vi "Sample - Job Record (SubVI).vi"(8 "error in":errorcluster) -> (0 "error out":errorcluster)   [LabVIEW 2019]
uses:
  Controls/Job record-state.ctl
  Controls/JSON - Job.ctl
  <vilib>/httpClient/POSTBuffer.vi
  <vilib>/httpClient/LabVIEWHTTPClient.lvlib
panel:
  in  "Please select Job No to delete":u16(ring) items=["GS1", "GS2"]
  in  "Ok":bool
  in  "Delete":bool
  out "TABLE":string[][](table)
  in  "Add":bool
  in  "Job Description":string
  in  "Job No":string
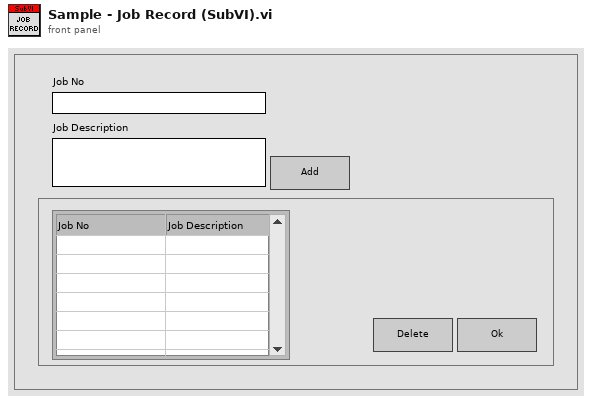
[diagram p1: front panel]
types:
  T1 = typedef "Job record-state.ctl" = enum16{"Init", "Read DB", "Idle", "update", "delete", "close"}
  T2 = typedef "JSON - Job.ctl" = cluster{"status":string, "data":cluster{"id":string, "jobno":string, "jobdesc":string, "delete":string, "created_date":string}[]}
  T3 = cluster{"action":string, "jobno":string, "jobdesc":string}
  T4 = cluster{"Jobs No":string, "Key Value":string[]}[]
  T5 = typedef "LabVIEWHTTPClient.lvlib/ClientHandle.ctl" = refnum<k1>
  T6 = cluster{"id":string, "jobno":string, "jobdesc":string, "delete":string, "created_date":string}[]
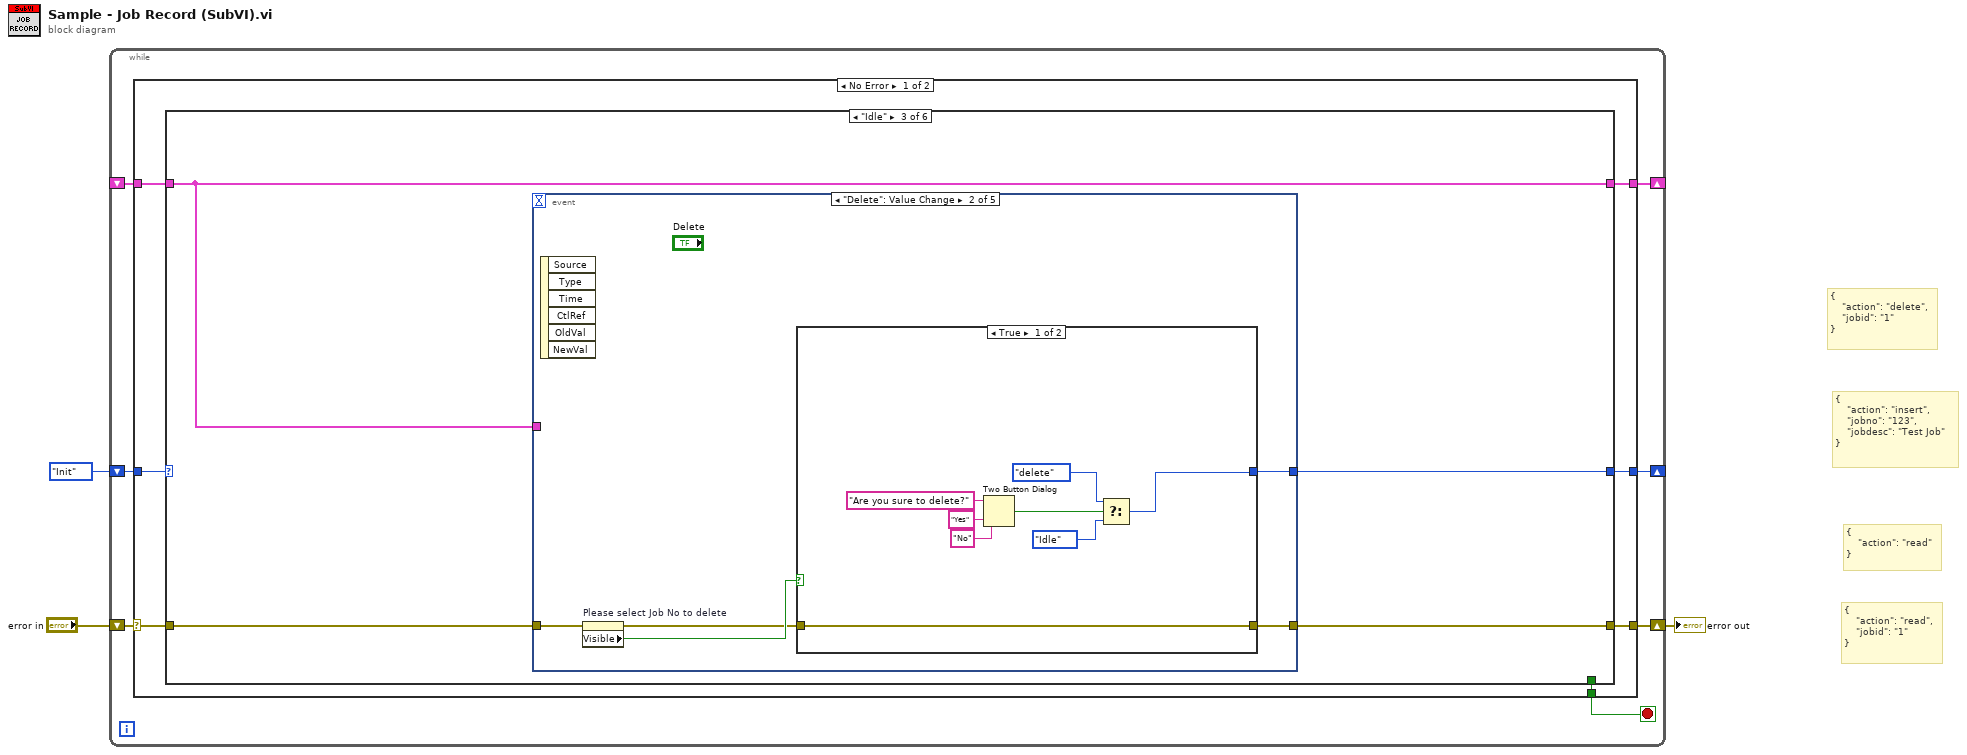
[diagram p0: block diagram]
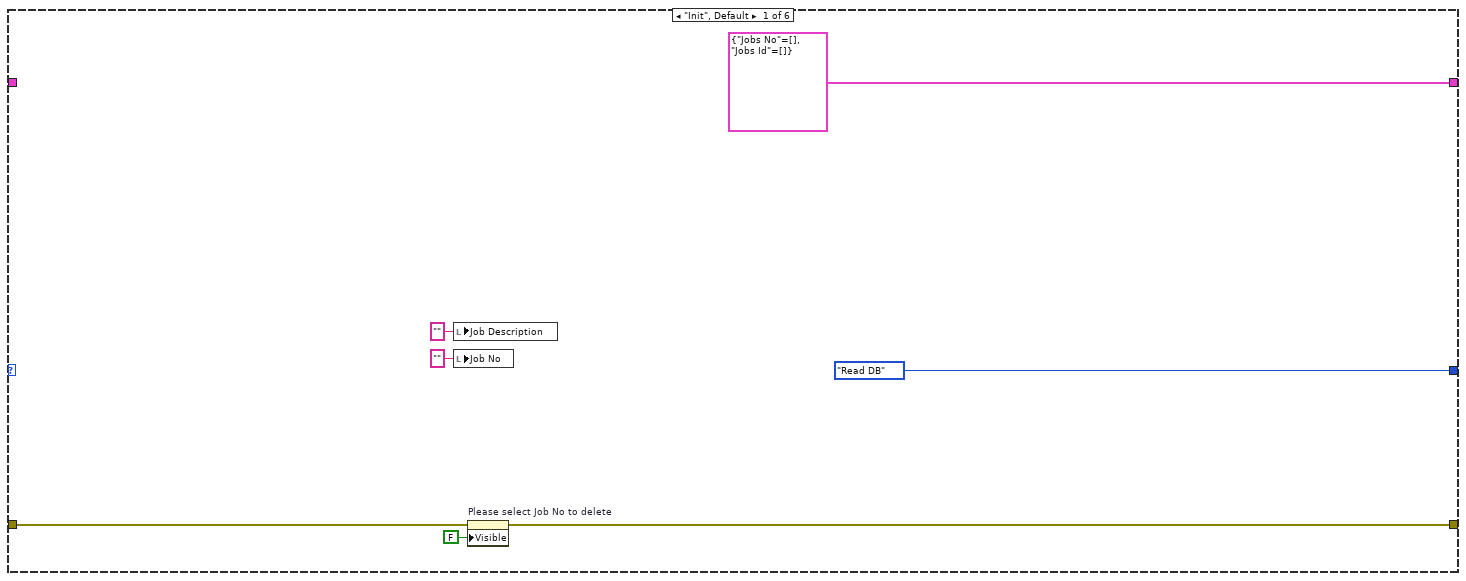
[diagram p2: hidden frame]
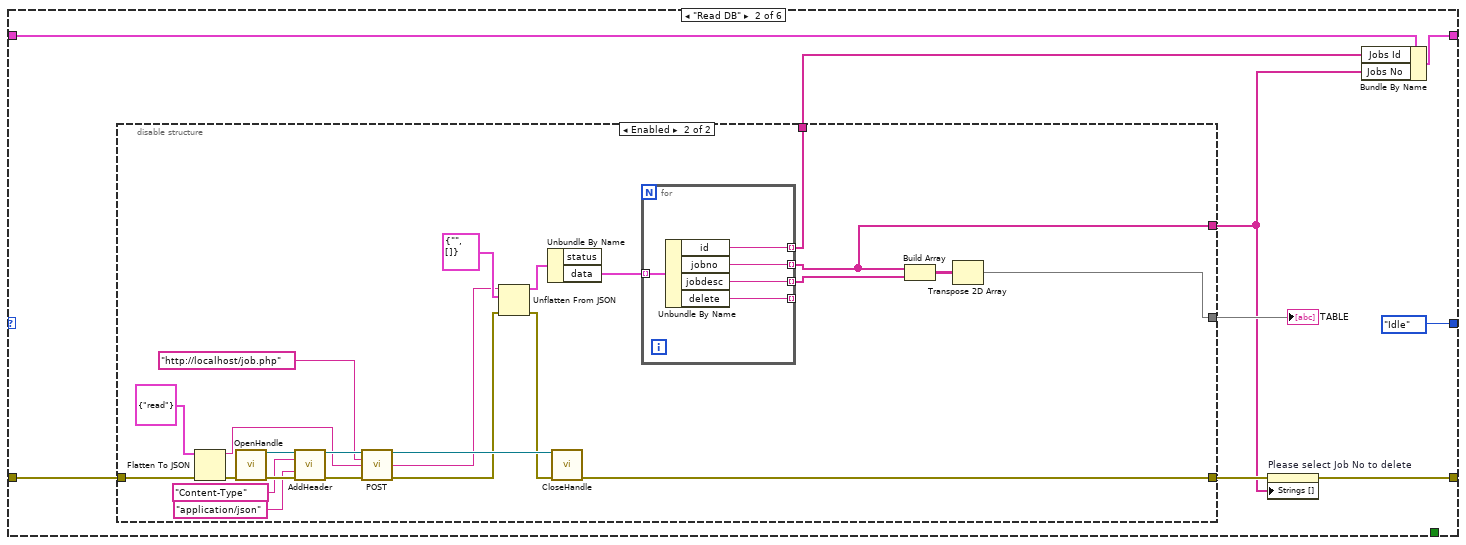
[diagram p3: hidden frame]
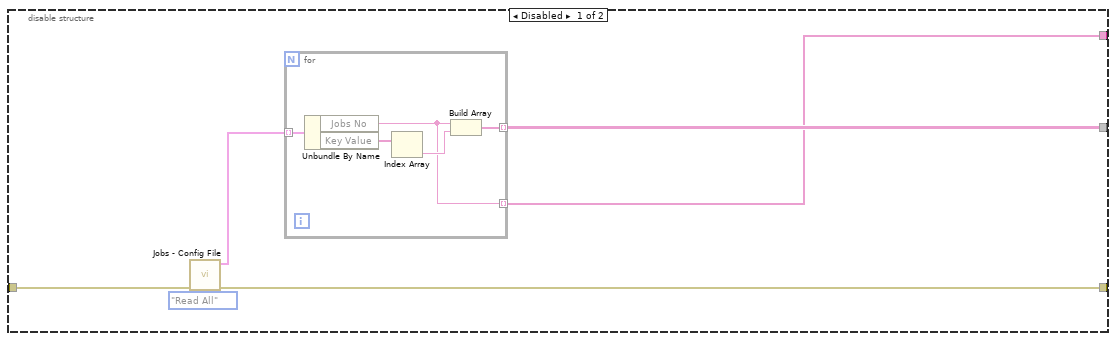
[diagram p4: hidden frame]
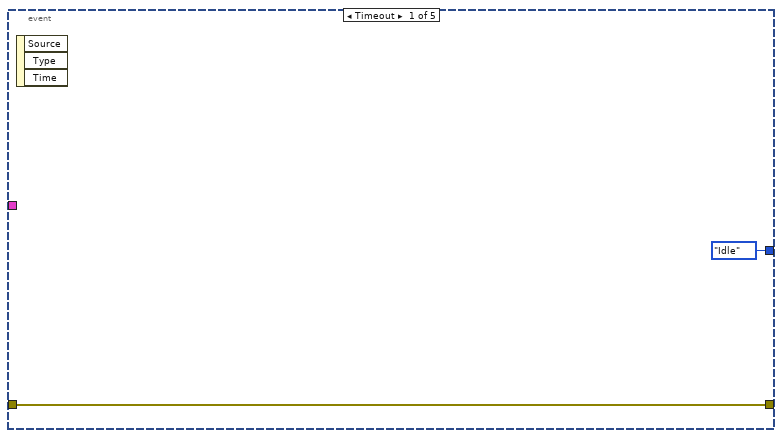
[diagram p5: hidden frame]
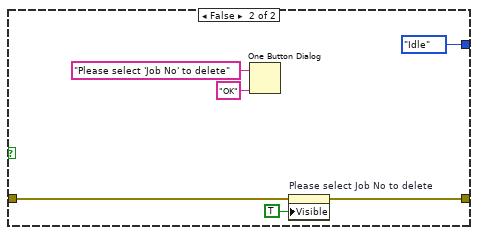
[diagram p6: hidden frame]
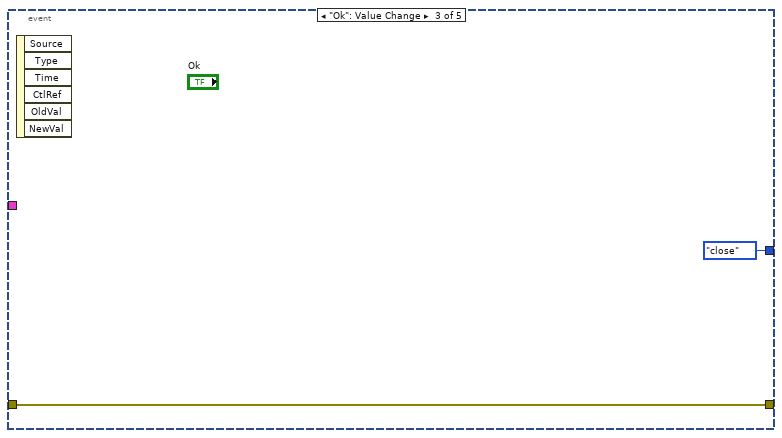
[diagram p7: hidden frame]
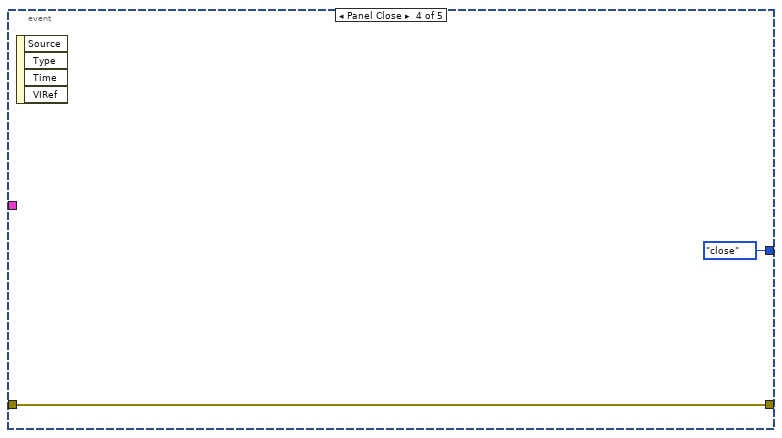
[diagram p8: hidden frame]
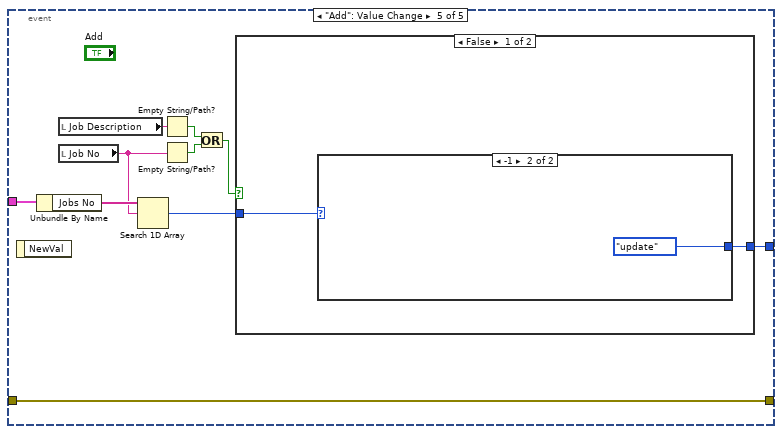
[diagram p9: hidden frame]
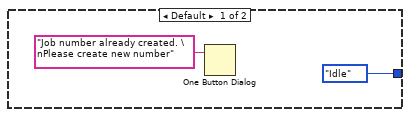
[diagram p10: hidden frame]
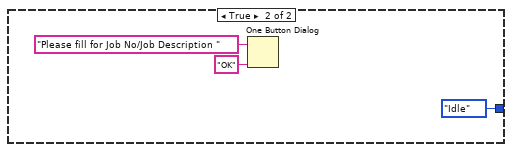
[diagram p11: hidden frame]
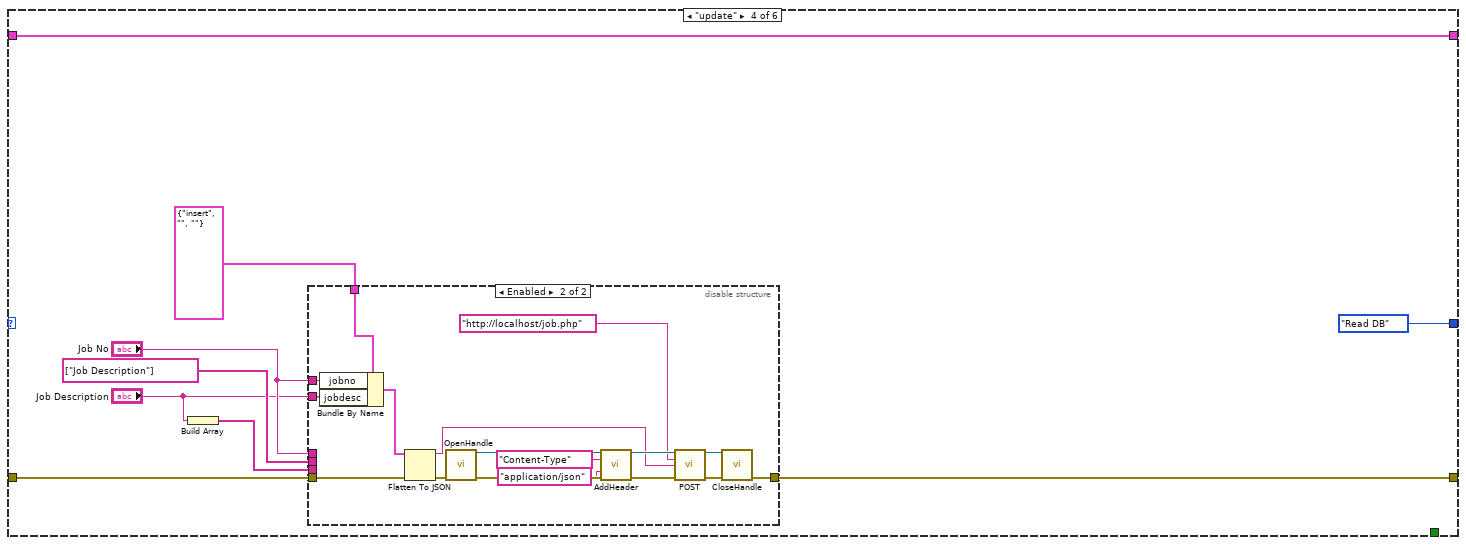
[diagram p12: hidden frame]
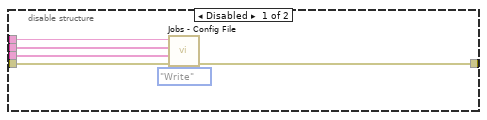
[diagram p13: hidden frame]
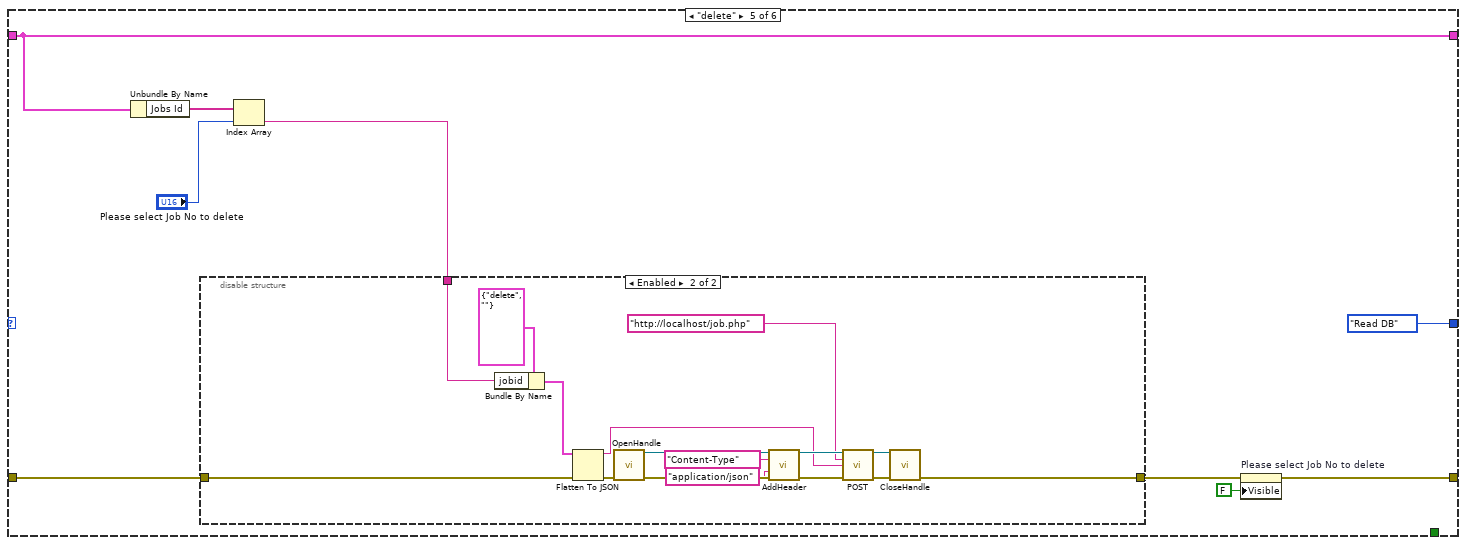
[diagram p14: hidden frame]
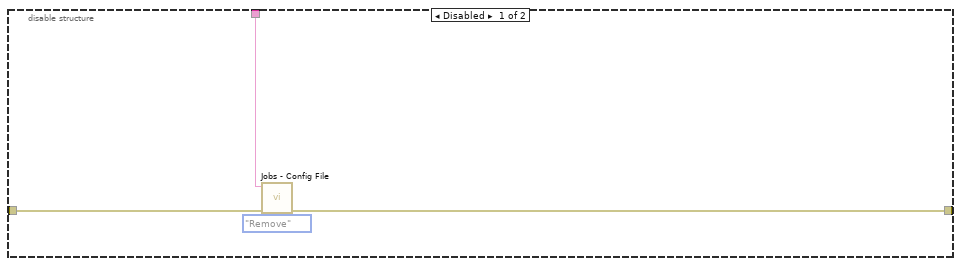
[diagram p15: hidden frame]
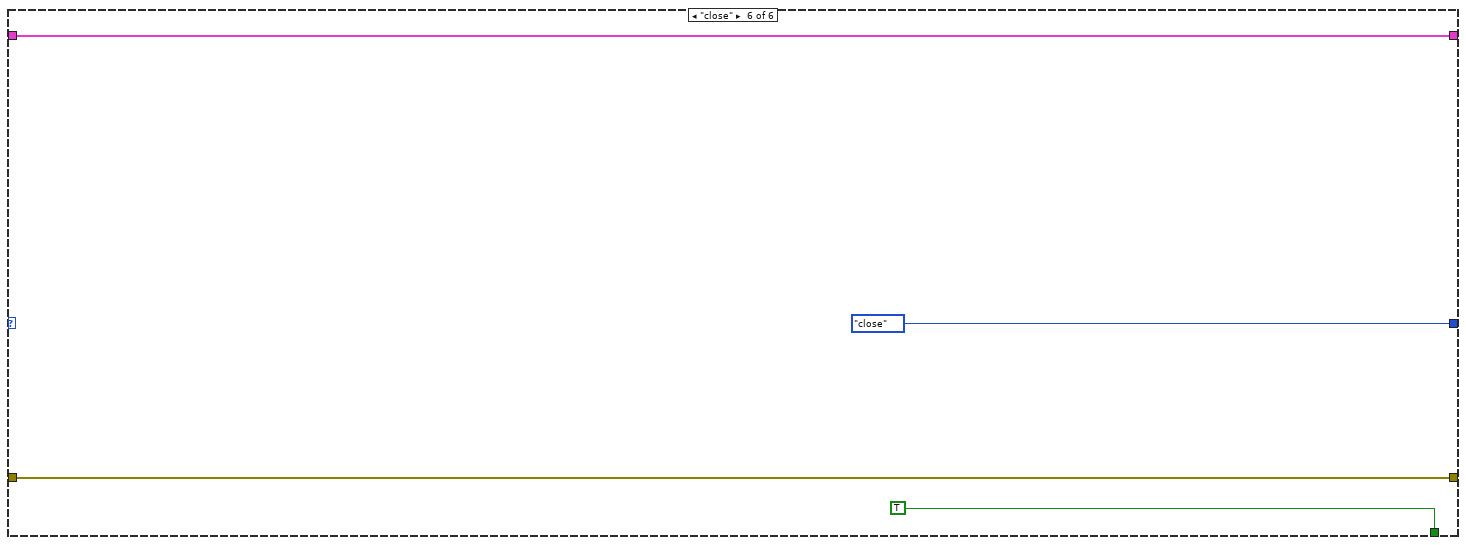
[diagram p16: hidden frame]
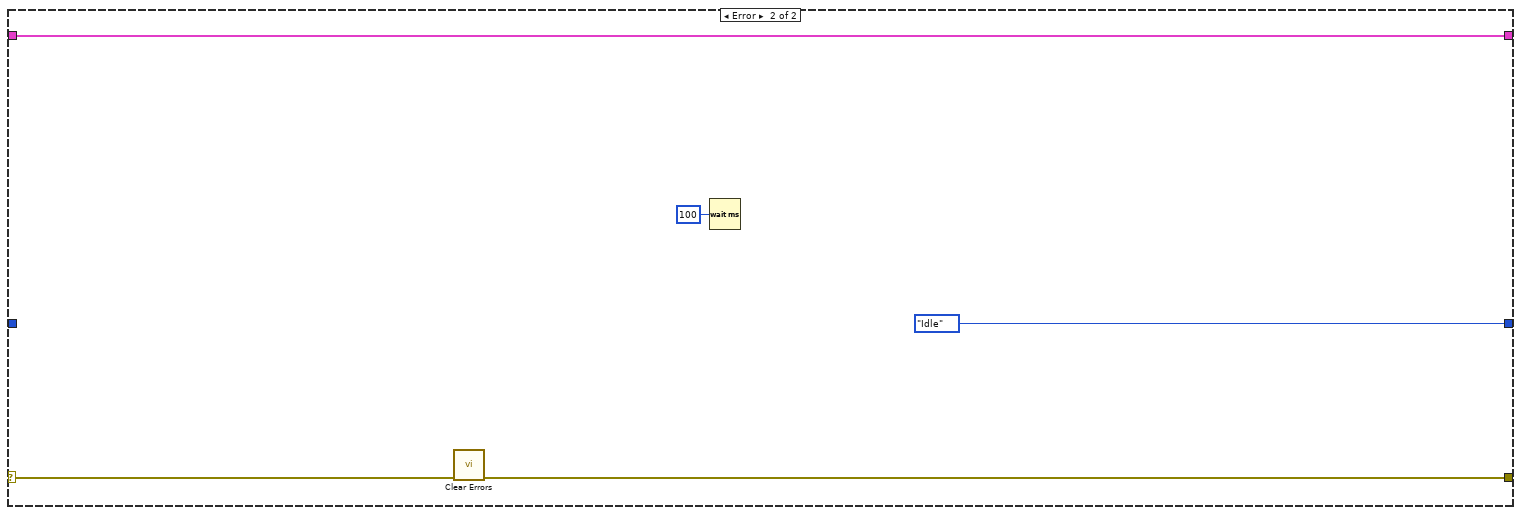
[diagram p17: hidden frame]
diagram:
  # "{\n    \"action\": \"read\",\n    \"jobid\": \"1\"\n}"
  # "{\n    \"action\": \"read\"\n}"
  # "{\n    \"action\": \"delete\",\n    \"jobid\": \"1\"\n}"
  # "{\n    \"action\": \"insert\",\n    \"jobno\": \"123\",\n    \"jobdesc\": \"Test Job\"\n}"
  n1 = while {
    shift-right: [w8] -> w1
    shift-left: "error in" -> [w10]
    shift-right: [w7] -> _
    shift-left: Job_record-state."Init" -> [w9]
    shift-right: [w6] -> _
    shift-left: _ -> [w5]
    stop <- w4 stop-if-true
    n2 = case shown="No Error" w10 {
      selector: w10 -> [w17 w190]
      tunnel: w9 -> [w16 _]
      tunnel: [w15 w189] -> w8
      tunnel: [w14 Job_record-state."Idle"] -> w7
      tunnel: [w13 w186] -> w6
      tunnel: w5 -> [w12 w186]
      tunnel: [w11 _] -> w4
      frame No Error {
        n3 = case shown="\"Idle\"" w16 {
          tunnel: w17 -> [w18 w30 w77 w127 w155 w185]
          tunnel: [w19 w28 w76 w126 w157 w185] -> w15
          tunnel: [Job_record-state."Read DB" Job_record-state."Idle" w75 Job_record-state."Read DB" Job_record-state."Read DB" Job_record-state."close"] -> w14
          tunnel: [cluster{"Jobs No":string[], "Jobs Id":string[]} {"Jobs No"=[], "Jobs Id"=[]} w32 w74 w128 w161 w182] -> w13
          tunnel: w12 -> [_ w31 w74 w128 w161 w182]
          tunnel: [_ _ _ _ _ TRUE] -> w11
          frame "Init", Default {
            n4 = local write "Job Description"("" ("Job Description")) -> ()
            n5 = local write "Job No"("" ("Job No")) -> ()
            n6 = property on="Please select Job No to delete" class="Ring (strict)"(error in=w18, "Visible"=FALSE) -> (error out=w19:errorcluster)  [unwired: 1 in, 1 out]
          }
          frame "Read DB" {
            n7 = disable-structure shown="Enabled" {
              disable-tunnel: w30 -> [w38 w58]
              disable-tunnel: [w36 w57] -> w29
              disable-tunnel: [w35 w47] -> w27
              disable-tunnel: [w34 w45] -> w26
              disable-tunnel: [_ w46] -> w25
              frame Disabled {
                n8 = call "Jobs - Config File.vi"("Action"=enum16{"Write", "Read", "Read All", "Remove"}."Read All", "error in (no error)"=w38) -> ("error out"=w36:errorcluster, "Value Out"=w37:T4)  [unwired: 7 in, 1 out]
                n9 = for {
                  tunnel: w37 -> [w44] mode=indexing
                  tunnel: [w41] -> w35 mode=indexing
                  tunnel: [w40] -> w34 mode=indexing
                  n10 = Unbundle By Name(w44) -> ("Jobs No"=w40:string, "Key Value"=w43:string[])
                  n11 = Index Array(array=w43) -> (element=w42:string)  [unwired: 1 in]
                  n12 = Build Array(w40, w42) -> (w41:string[])
                }
              }
              frame Enabled {
                n13 = Flatten To JSON(anything=cluster{"action":string} {"action"="read"}, error in (no error)=w58) -> (JSON string=w62:string, 11:w63:errorcluster)  [unwired: 1 in]
                n14 = call <vilib>:"OpenHandle.vi"("error in (no error)"=w63) -> ("client handle out"=w66:T5, "error out"=w68:errorcluster)  [unwired: 13 in]
                n15 = call <vilib>:"AddHeader.vi"("client handle"=w66, "header"="Content-Type", "value"="application/json", "error in (no error)"=w68) -> ("client handle out"=w65:T5, "error out"=w67:errorcluster)  [unwired: 10 in]
                n16 = call-poly <vilib>:"POST.vi"("client handle"=w65, "url"="http://localhost/job.php", "buffer"=w62, "error in (no error)"=w67) -> ("client handle out"=w64:T5, "body"=w52:string, "error out"=w51:errorcluster)  [unwired: 8 in, 1 out]
                n17 = Unflatten From JSON(JSON string=w52, type and defaults=T2 {"status"="", "data"=[]}, error in (no error)=w51) -> (value=w54:T2, error out=w50:errorcluster)  [unwired: 4 in]
                n18 = Unbundle By Name(w54) -> ("data"=w53:T6)  [unwired: 1 out]
                n19 = call <vilib>:"CloseHandle.vi"("client handle"=w64, "error in (no error)"=w50) -> ("error out"=w57:errorcluster)  [unwired: 13 in]
                n20 = for {
                  tunnel: w53 -> [w73] mode=indexing
                  tunnel: [w72] -> w46 mode=indexing
                  tunnel: [w71] -> w45 mode=indexing
                  tunnel: [w70] -> w49 mode=indexing
                  tunnel: [w69] -> _ mode=indexing
                  n21 = Unbundle By Name(w73) -> ("id"=w72:string, "jobno"=w71:string, "jobdesc"=w70:string, "delete"=w69:string)
                }
                n22 = Build Array(w45, w49) -> (w48:string[][])
                n23 = Transpose 2D Array(2D array=w48) -> (transposed array=w47:string[][])
              }
            }
            "TABLE" <- w27
            n24 = property on="Please select Job No to delete" class="Ring (strict)"(error in=w29, "Strings []"=w26) -> (error out=w28:errorcluster)  [unwired: 1 in, 1 out]
            n25 = Bundle By Name(cluster=w31, "Jobs Id"=w25, "Jobs No"=w26) -> (w32:cluster{"Jobs No":string[], "Jobs Id":string[]})
          }
          frame "Idle" {
            n26 = event shown="[1] \"Delete\": Value Change" {
              selector: _ -> [_ _ _ _ _]
              dyn-events: _ -> [_ _ _ _ _]
              timeout: _ -> [_ _ _ _ _]
              tunnel: [w79 w82 w99 w101 w112] -> w76
              tunnel: w77 -> [w79 w80 w99 w101 w112]
              tunnel: [Job_record-state."Idle" w84 Job_record-state."close" Job_record-state."close" w111] -> w75
              tunnel: w74 -> [_ _ _ _ w106]
              event Timeout {
                n27 = event-data() -> ()  [unwired: 1 in, 3 out]
              }
              event "Delete": Value Change {
                n28 = event-data() -> ()  [unwired: 1 in, 6 out]
                n29 = property on="Please select Job No to delete" class="Ring (strict)"(error in=w80) -> (error out=w81:errorcluster, "Visible"=w83:bool)  [unwired: 1 in, 1 out]
                n30 = case shown="True" w83 {
                  tunnel: [w87 Job_record-state."Idle"] -> w84
                  tunnel: w81 -> [w85 w96]
                  tunnel: [w85 w95] -> w82
                  frame True {
                    n31 = Two Button Dialog(message="Are you sure to delete?", 1:"No" ("F button name (\"Cancel\")"), 2:"Yes" ("T button name (\"OK\")")) -> (T button?=w89:bool)
                    n32 = Select(t=Job_record-state."delete", s=w89, f=Job_record-state."Idle") -> (s? t:f=w87:T1)
                  }
                  frame False {
                    n33 = One Button Dialog(message="Please select 'Job No' to delete", button name ("OK")="OK") -> ()  [unwired: 1 out]
                    n34 = property on="Please select Job No to delete" class="Ring (strict)"(error in=w96, "Visible"=TRUE) -> (error out=w95:errorcluster)  [unwired: 1 in, 1 out]
                  }
                }
              }
              event "Ok": Value Change {
                n35 = event-data() -> ()  [unwired: 1 in, 6 out]
              }
              event Panel Close {
                n36 = event-data() -> ()  [unwired: 1 in, 4 out]
              }
              event "Add": Value Change {
                n37 = event-data() -> ()  [unwired: 1 in, 1 out]
                n38 = Unbundle By Name(w106) -> ("Jobs No"=w105:string[])
                n39 = local read "Job Description"() -> (w110:string)
                n40 = local read "Job No"() -> (w104:string)
                n41 = Search 1D Array(1D array=w105, element=w104) -> (index of element=w103:i32)  [unwired: 1 in]
                n42 = Empty String/Path?(string/path=w110) -> (empty?=w109:bool)
                n43 = Empty String/Path?(string/path=w104) -> (empty?=w108:bool)
                n44 = Or(x=w109, y=w108) -> (x .or. y?=w107:bool)
                n45 = case shown="False" w107 {
                  tunnel: [w114 Job_record-state."Idle"] -> w111
                  tunnel: w103 -> [w113 _]
                  frame False {
                    n46 = case shown="-1" w113 {
                      tunnel: [Job_record-state."Idle" Job_record-state."update"] -> w114
                      frame Default {
                        n47 = One Button Dialog(message="Job number already created. \nPlease create new number") -> ()  [unwired: 1 in, 1 out]
                      }
                      frame -1 {
                      }
                    }
                  }
                  frame True {
                    n48 = One Button Dialog(message="Please fill for Job No/Job Description ", button name ("OK")="OK") -> ()  [unwired: 1 out]
                  }
                }
              }
            }
          }
          frame "update" {
            n49 = Build Array("Job Description") -> (w124:string[])
            n50 = disable-structure shown="Enabled" {
              disable-tunnel: w127 -> [w135 w141]
              disable-tunnel: [w134 w144] -> w126
              disable-tunnel: "Job No" -> [w132 _]
              disable-tunnel: string[] ["Job Description"] ("Key Name") -> [w131 _]
              disable-tunnel: w124 -> [w130 _]
              disable-tunnel: T3 {"action"="insert", "jobno"="", "jobdesc"=""} -> [_ w140]
              disable-tunnel: "Job No" -> [_ w139]
              disable-tunnel: "Job Description" -> [_ w138]
              frame Disabled {
                n51 = call "Jobs - Config File.vi"("Action"=enum16{"Write", "Read", "Read All", "Remove"}."Write", "error in (no error)"=w135, "Value"=w130, "Key Name"=w131, "Jobs No"=w132) -> ("error out"=w134:errorcluster)  [unwired: 4 in, 2 out]
              }
              frame Enabled {
                n52 = Bundle By Name(cluster=w140, "jobno"=w139, "jobdesc"=w138) -> (w137:T3)
                n53 = Flatten To JSON(anything=w137, error in (no error)=w141) -> (JSON string=w136:string, 11:w142:errorcluster)  [unwired: 1 in]
                n54 = call <vilib>:"OpenHandle.vi"("error in (no error)"=w142) -> ("client handle out"=w150:T5, "error out"=w152:errorcluster)  [unwired: 13 in]
                n55 = call <vilib>:"AddHeader.vi"("client handle"=w150, "header"="Content-Type", "value"="application/json", "error in (no error)"=w152) -> ("client handle out"=w149:T5, "error out"=w151:errorcluster)  [unwired: 10 in]
                n56 = call-poly <vilib>:"POST.vi"("client handle"=w149, "url"="http://localhost/job.php", "buffer"=w136, "error in (no error)"=w151) -> ("client handle out"=w143:T5, "error out"=w145:errorcluster)  [unwired: 8 in, 2 out]
                n57 = call <vilib>:"CloseHandle.vi"("client handle"=w143, "error in (no error)"=w145) -> ("error out"=w144:errorcluster)  [unwired: 13 in]
              }
            }
          }
          frame "delete" {
            n58 = Unbundle By Name(w161) -> ("Jobs Id"=w160:string[])
            n59 = Index Array(array=w160, index="Please select Job No to delete") -> (element=w153:string)
            n60 = disable-structure shown="Enabled" {
              disable-tunnel: w155 -> [w164 w168]
              disable-tunnel: [w163 w167] -> w154
              disable-tunnel: w153 -> [w162 w166]
              frame Disabled {
                n61 = call "Jobs - Config File.vi"("Action"=enum16{"Write", "Read", "Read All", "Remove"}."Remove", "error in (no error)"=w164, "Jobs No"=w162) -> ("error out"=w163:errorcluster)  [unwired: 6 in, 2 out]
              }
              frame Enabled {
                n62 = Bundle By Name(cluster=cluster{"action":string, "jobid":string} {"action"="delete", "jobid"=""}, "jobid"=w166) -> (w170:cluster{"action":string, "jobid":string})
                n63 = Flatten To JSON(anything=w170, error in (no error)=w168) -> (JSON string=w169:string, 11:w171:errorcluster)  [unwired: 1 in]
                n64 = call <vilib>:"OpenHandle.vi"("error in (no error)"=w171) -> ("client handle out"=w178:T5, "error out"=w180:errorcluster)  [unwired: 13 in]
                n65 = call <vilib>:"AddHeader.vi"("client handle"=w178, "header"="Content-Type", "value"="application/json", "error in (no error)"=w180) -> ("client handle out"=w177:T5, "error out"=w179:errorcluster)  [unwired: 10 in]
                n66 = call-poly <vilib>:"POST.vi"("client handle"=w177, "url"="http://localhost/job.php", "buffer"=w169, "error in (no error)"=w179) -> ("client handle out"=w172:T5, "error out"=w173:errorcluster)  [unwired: 8 in, 2 out]
                n67 = call <vilib>:"CloseHandle.vi"("client handle"=w172, "error in (no error)"=w173) -> ("error out"=w167:errorcluster)  [unwired: 13 in]
              }
            }
            n68 = property on="Please select Job No to delete" class="Ring (strict)"(error in=w154, "Visible"=FALSE) -> (error out=w157:errorcluster)  [unwired: 1 in, 1 out]
          }
          frame "close" {
          }
        }
      }
      frame Error {
        n69 = call <vilib>:"Clear Errors.vi"("error in (no error)"=w190) -> ("error out"=w189:errorcluster)  [unwired: 5 in, 1 out]
        n70 = Wait (ms)(milliseconds to wait=u32 100) -> ()  [unwired: 1 out]
      }
    }
  }
  "error out" <- w1
